vi "Subvi counter up stop U16.vi"(4 "Reset":bool, 6 "Gating":bool, 9 "Clock":bool) -> (1 "Output":u16)   [LabVIEW 2017]
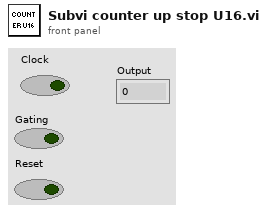
[diagram p1: front panel]
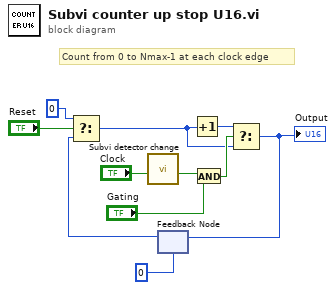
[diagram p0: block diagram]
diagram:
  # "Count from 0 to Nmax-1 at each clock edge"
  n1 = call "Subvi detector change.vi"("Input"="Clock") -> ("Output"=w7:bool)  [unwired: 8 in]
  n2 = feedback #1(u16 0) -> (w2:u16)
  n3 = Select(t=u16 0, s="Reset", f=w2) -> (s? t:f=w3:u16)
  n4 = Increment(x=w3) -> (x+1=w8:u16)
  n5 = And(x=w7, y="Gating") -> (x .and. y?=w6:bool)
  n6 = Select(t=w8, s=w6, f=w3) -> (s? t:f=w10:u16)
  "Output" <- w10
  n7 = feedback-in #1(w10) -> ()
